vi "RS232 S&R.vi"(0 "ReSetSP":bool, 4 "Speed":cluster{"Speed":i32, "Vi":i32, "Vi steps":i32}={"Speed"=3111, "Vi"=1000, "Vi steps"=800} {"Speed" min=50 max=8000 step=50 scale=50.0..8000.0}, 5 "Delay (ms)":u32, 6 "error in":errorcluster, 7 "Read":bool, 8 "write buffer":string="r", 9 "VISA resource in":refnum<visa-resource-name>) -> (1 "read buffer":string, 2 "error out":errorcluster, 3 "VISA resource name out":refnum<visa-resource-name>)   [LabVIEW 2014]
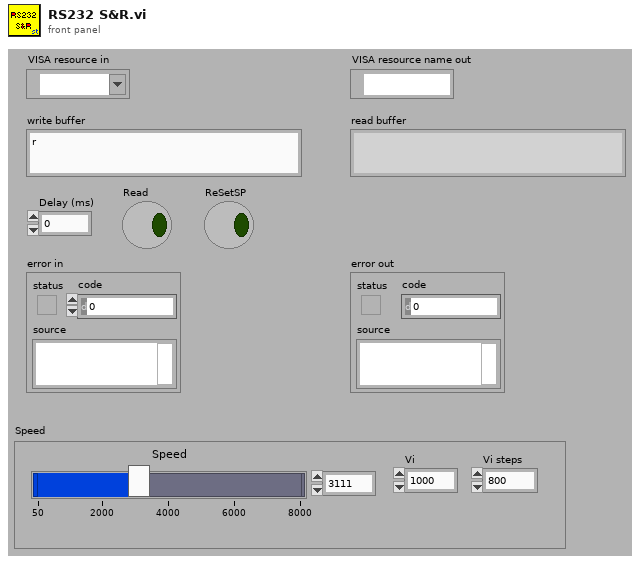
[diagram p1: front panel]
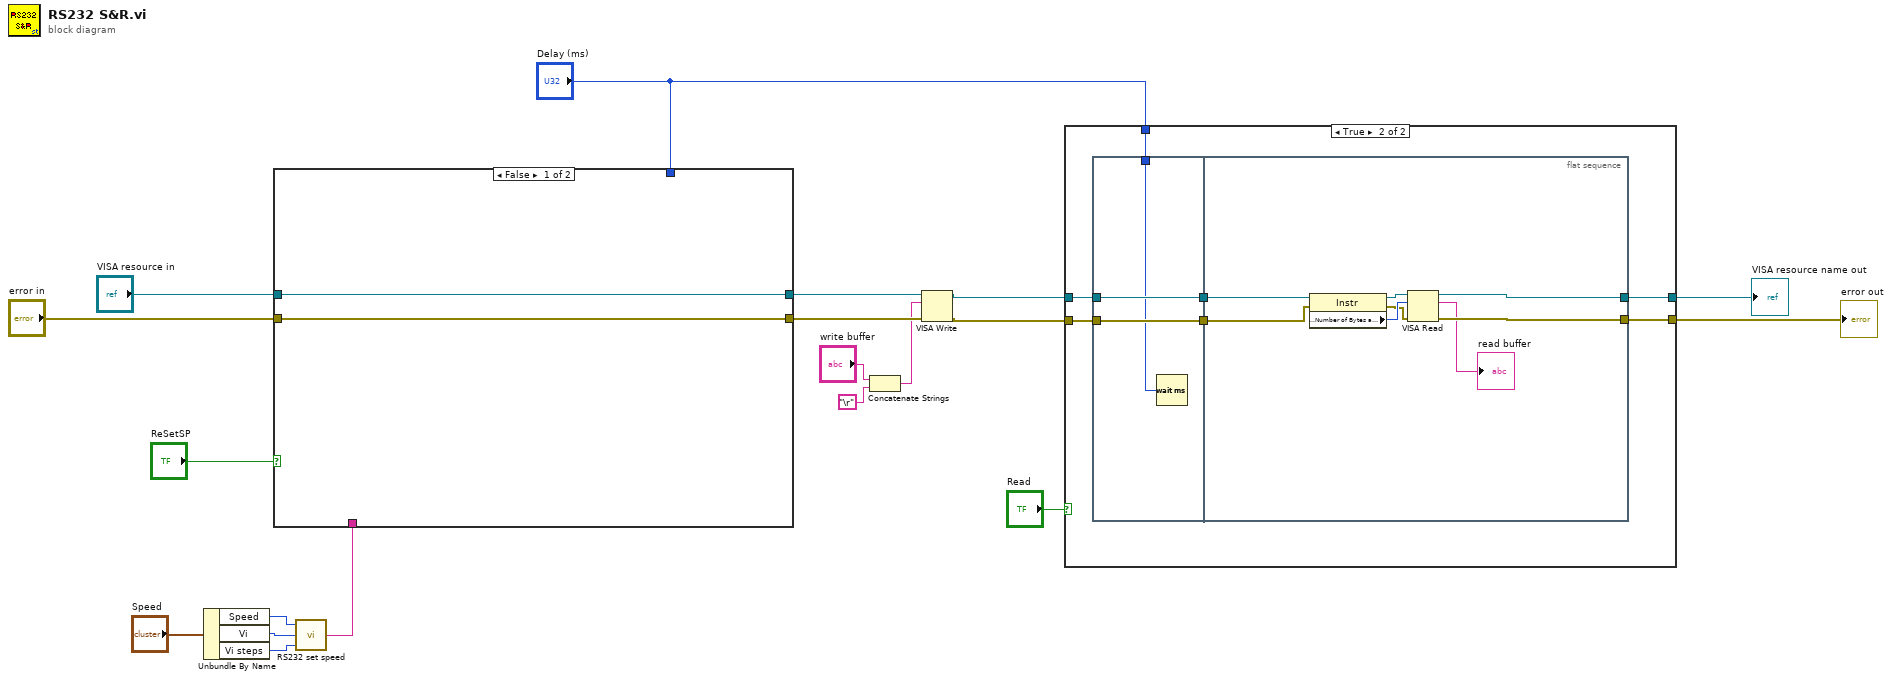
[diagram p0: block diagram]
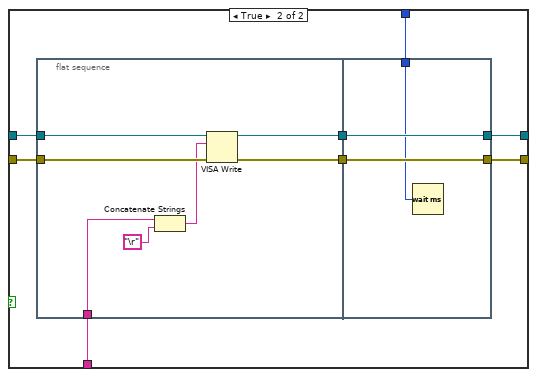
[diagram p2: hidden frame]
diagram:
  n1 = Unbundle By Name("Speed") -> ("Speed"=w12:i32, "Vi"=w13:i32, "Vi steps"=w14:i32)
  n2 = call "RS232 set speed.vi"("Vi steps"=w14, "Vi"=w13, "Speed"=w12) -> ("Command"=w8:string)
  n3 = case shown="False" "ReSetSP" {
    tunnel: "VISA resource in" -> [w21 w27]
    tunnel: "error in" -> [w20 w26]
    tunnel: w8 -> [_ w25]
    tunnel: [w21 w24] -> w7
    tunnel: [w20 w23] -> w6
    tunnel: "Delay (ms)" -> [_ w22]
    frame False {
    }
    frame True {
      n4 = flat-sequence {
        tunnel: w27 -> [w36]
        tunnel: w26 -> [w35]
        tunnel: w25 -> [w34]
        tunnel: [w33] -> w29
        tunnel: [w32] -> w28
        tunnel: [w38] -> w23
        tunnel: [w39] -> w24
        tunnel: w29 -> [w39]
        tunnel: w28 -> [w38]
        tunnel: w22 -> [w37]
        frame #0 {
          n5 = Concatenate Strings(w34, "\r") -> (w31:string)
          n6 = VISA Write(VISA resource name=w36, write buffer=w31, error in (no error)=w35) -> (VISA resource name out=w33:refnum<visa-resource-name>, error out=w32:errorcluster)  [unwired: 1 out]
        }
        frame #1 {
          n7 = Wait (ms)(milliseconds to wait=w37) -> ()  [unwired: 1 out]
        }
      }
    }
  }
  n8 = Concatenate Strings("write buffer", "\r") -> (w5:string)
  n9 = VISA Write(VISA resource name=w7, write buffer=w5, error in (no error)=w6) -> (VISA resource name out=w17:refnum<visa-resource-name>, error out=w16:errorcluster)  [unwired: 1 out]
  n10 = case shown="True" "Read" {
    tunnel: [w40 w46] -> w19
    tunnel: [w41 w45] -> w18
    tunnel: w17 -> [w41 w44]
    tunnel: w16 -> [w40 w43]
    tunnel: "Delay (ms)" -> [_ w42]
    frame False {
    }
    frame True {
      n11 = flat-sequence {
        tunnel: w43 -> [w50]
        tunnel: w44 -> [w51]
        tunnel: [w51] -> w48
        tunnel: [w50] -> w47
        tunnel: w42 -> [w49]
        tunnel: [w59] -> w46
        tunnel: [w58] -> w45
        tunnel: w48 -> [w57]
        tunnel: w47 -> [w56]
        frame #0 {
          n12 = Wait (ms)(milliseconds to wait=w49) -> ()  [unwired: 1 out]
        }
        frame #1 {
          n13 = property class="Instr"(reference=w57, error in=w56) -> (reference out=w55:refnum<visa-resource-name>, error out=w52:errorcluster, "Serial Settings:Number of Bytes at Serial Port"=w53:u32)
          n14 = VISA Read(VISA resource name=w55, byte count=w53, error in (no error)=w52) -> (VISA resource name out=w58:refnum<visa-resource-name>, read buffer=→"read buffer":string, error out=w59:errorcluster)  [unwired: 1 out]
        }
      }
    }
  }
  "error out" <- w19
  "VISA resource name out" <- w18
